vi "Caching_Expression_Evaluator_v4.vi"(0 "method":T1, 5 "variable":string, 7 "value in":dbl, 9 "expression/scriptlet":string, 11 "error in (no error)":errorcluster) -> (8 "value out":dbl, 15 "error out":errorcluster)   [LabVIEW 2013]
doc: "This \"object\" caches variables and parsed expressions for fast evaluation and assignment. It is possible to {set} or {get} a variable, {eval}uate an expression, or evaluate and {assign} an expression to a variable. The {isvalid} method tests whether a variable name is a valid identifier and does not collide with one of the predefined functions or numbers. To set initial values or define custom functions, {execute} a scriptlet.\n\nExpressions and scriptlets can make use Lua's arithmetic operators, the predefined numerical values \"pi\", \"_NaN\", and \"_Inf\", the functions in the math library (sin(), sqrt(), etc.) and the lv library functions for bitwise and other integer operations (andU32(), addI8(), etc.). To promote compact expressions, both sets of functions are available only without their library (\"math.\", \"lv.\") table prefix."
uses:
  t_Caching_Expression_Evaluator_Methods_v4.ctl
  LuaVIEW1.2.2_full_LV85/luaview/subvis/private/LuaVIEW Push (string).vi
  LuaVIEW1.2.2_full_LV85/luaview/subvis/private/LuaVIEW Push (number).vi
  LuaVIEW1.2.2_full_LV85/luaview/subvis/private/LuaVIEW Pull (number).vi
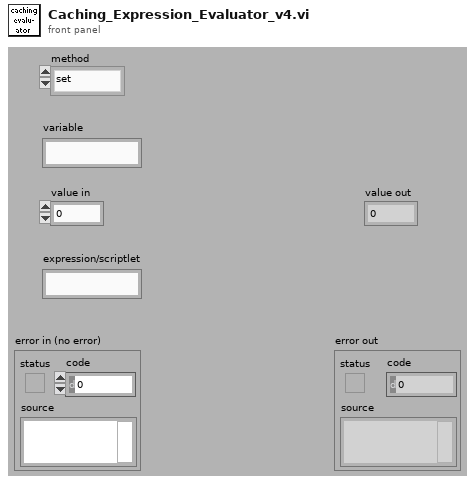
[diagram p1: front panel]
types:
  T1 = typedef "t_Caching_Expression_Evaluator_Methods_v4.ctl" = enum16{"set", "get", "eval", "eval2", "assign", "execute", "isvalid"}
  T2 = typedef "t_LuaVIEW Reference.ctl" = refnum<k1>
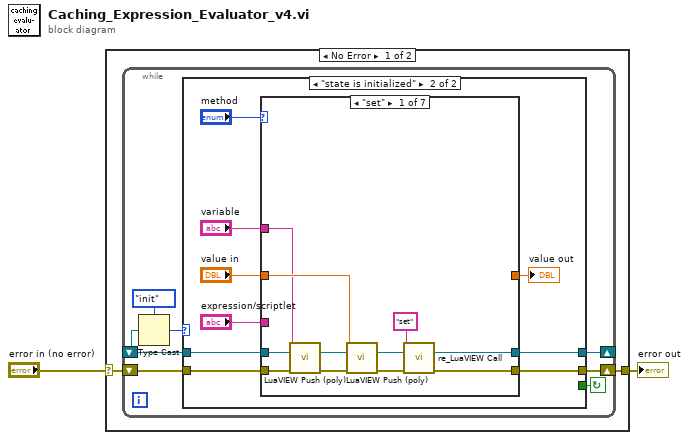
[diagram p0: block diagram]
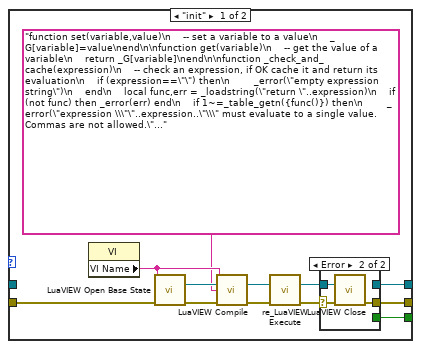
[diagram p2: hidden frame]
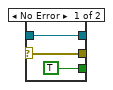
[diagram p3: hidden frame]
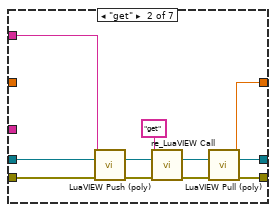
[diagram p4: hidden frame]
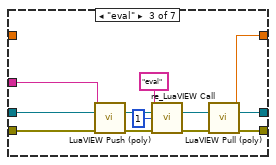
[diagram p5: hidden frame]
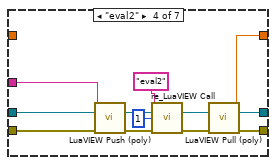
[diagram p6: hidden frame]
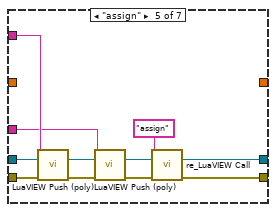
[diagram p7: hidden frame]
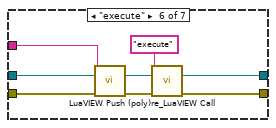
[diagram p8: hidden frame]
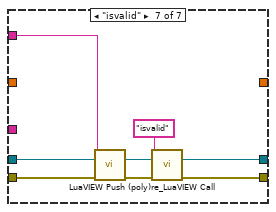
[diagram p9: hidden frame]
diagram:
  n1 = case shown="No Error" "error in (no error)" {
    selector: "error in (no error)" -> [w3 w112]
    tunnel: [w4 w112] -> w1
    frame No Error {
      n2 = while {
        shift-right: [w10] -> _
        shift-left: _ -> [w8]
        shift-right: [w9] -> w4
        shift-left: w3 -> [w11]
        stop <- w5 continue-if-true
        n3 = Type Cast(type=enum32{"init", "state is initialized"}."init", x=w8) -> (*(type *) &x=w6:enum32{"init", "state is initialized"})
        n4 = case shown="\"state is initialized\"" w6 {
          tunnel: w11 -> [w23 w38]
          tunnel: [w13 w35] -> w10
          tunnel: [w14 w36] -> w9
          tunnel: w8 -> [_ w37]
          tunnel: [w12 _] -> w5
          frame "init" {
            n5 = property class="VI"() -> ("VI Name"=w19:string)  [unwired: 2 in, 2 out]
            n6 = call "LuaVIEW Open Base State.vi"("close identifier (none)"=w19, "error in (no error)"=w23) -> ("LuaVIEW reference"=w21:T2, "error out"=w17:errorcluster)  [unwired: 12 out]
            n7 = call "LuaVIEW Compile.vi"("script name"=w19, "LuaVIEW reference in"=w21, "script"="function set(variable,value)\n    -- set a variable to a value\n    _G[variable]=value\nend\n\nfunction get(variable)\n    -- get the value of a variable\n    return _G[variable]\nend\n\nfunction _check_and_cache(expression)\n    -- check an expression, if OK cache it and return its evaluation\n    if (expression==\"\") then\n        _error(\"empty expression string\")\n    end\n    local func,err = _loadstring(\"return \"..expression)\n    if (not func) then _error(err) end\n    if 1~=_table_getn({func()}) then\n        _error(\"expression \\\"\"..expression..\"\\\" must evaluate to a single value. Commas are not allowed.\")\n    end\n    local result=func()\n    if _type(result)~=\"number\" then\n        _error(\"expression \\\"\"..expression..\"\\\" does not evaluate to a number\")\n    end\n    _expression_cache[expression]=func\n    return result\nend\n\nfunction eval(expression)\n    -- evaluate an expression and return its value\n    local func=_expression_cache[expression]\n    if (func) then\n        -- expression already parsed and cached\n        return func()\n    end\n    return _check_and_cache(expression)\nend\n\n-- New code from IBS\n-- Eval didn't work with my custom functions\nfunction eval2(expression)\n    -- evaluate an expression and return its value\n    local func=_expression_cache[expression]\n    if (not func) then\n        -- expression not parsed and cached\n        _check_and_cache(expression)\n        func=_expression_cache[expression]\n    end\n    -- expression is now parsed and cached\n    -- now make the desired tabular evaluation\n    \n    local answer;\n\n    dt = 0.1;\n    tMax = 1;\n    t = 0;\n    f = 0.1;\n    answer = func()\n    \n    return answer\nend\n\n\nfunction assign(variable,expression)\n    -- evaluate an expression and assign it to a variable\n    local func=_expression_cache[expression]\n    if (func) then\n        -- expression already parsed and cached\n        _G[variable]=func()\n        return\n    end\n    _G[variable]=_check_and_cache(expression)\nend\n\nfunction execute(statements)\n    -- execute statements, e.g. setting initial variable values\n    -- or defining custom functions\n    local func,err=_loadstring(statements)\n    if (not func) then\n        _error(err)\n    end\n    func()\nend\n\nfunction isvalid(variable)\n    -- check if a variable name is valid for assignment\n    if _name_reserved[variable] then\n        _error(\"\\\"\"..variable..\"\\\" is not a valid variable name: it is reserved for a predefined \".._type(_G[variable]))\n    end\n    if _string_find(variable,\"[^_%w]\") then\n        _error(\"\\\"\"..variable..\"\\\" is not a valid variable name: only underscores and alphanumerical characters are allowed.\")\n    end\n    if (not _loadstring(\"return {\"..variable..\"=42}\")) then\n        _error(\"\\\"\"..variable..\"\\\" is not a valid variable name: leading digits and Lua reserved names are prohibited.\")\n    end    \nend\n\n--start with an empty expression cache\n_expression_cache={}\n\n-- hide functions and tables that do not belong in expressions\n_error=error\n_type=type\n_table_getn=table.getn\n_string_find=string.find\n_loadstring=loadstring\nretain={\nretain=true,\nset=true,\nget=true,\neval=true,\nassign=true,\nexecute=true,\nisvalid=true,\nstring=true,\nmath=true,\n}\nfor k,v in pairs(lv) do\n    if (string.find(k,\"I8\") or string.find(k,\"U8\") or string.find(k,\"I16\") or string.find(k,\"U16\") or string.find(k,\"I32\") or string.find(k,\"U32\")) then\n        _G[k]=v\n        retain[k]=true\n    end\nend\n_name_reserved={}\nfor k,v in pairs(_G) do\n    if _type(k)==\"string\" and not (retain[k] or math[k] or string.sub(k,1,1)==\"_\") then\n        _G[k]=nil\n    else\n        _name_reserved[k]=true\n    end\nend\nmath=nil\n_name_reserved.math=nil\nretain=nil\n_name_reserved.retain=nil\nstring=nil\n_name_reserved.string=nil\n\nf=0\nt=0\ntMax = 0\ndt = 0", "error in (no error)"=w17) -> ("LuaVIEW reference out"=w20:T2, "error out"=w22:errorcluster)  [unwired: 10 out]
            n8 = call "re_LuaVIEW Execute.vi"("LuaVIEW reference in"=w20, "error in (no error)"=w22) -> ("LuaVIEW reference out"=w15:T2, "error out"=w16:errorcluster)  [unwired: 12 out]
            n9 = case shown="Error" w16 {
              selector: w16 -> [w25 w29]
              tunnel: w15 -> [w26 w28]
              tunnel: [w25 w27] -> w14
              tunnel: [w26 _] -> w13
              tunnel: [TRUE _] -> w12
              frame No Error {
              }
              frame Error {
                n10 = call "LuaVIEW Close.vi"("LuaVIEW reference"=w28, "error in (no error)"=w29) -> ("dup error"=w27:errorcluster)  [unwired: 13 out]
              }
            }
          }
          frame "state is initialized" {
            n11 = case shown="\"set\"" "method" {
              tunnel: w38 -> [w46 w50 w62 w74 w92 w99 w106]
              tunnel: w37 -> [w47 w51 w63 w75 w93 w100 w107]
              tunnel: [w39 w60 w72 w84 w85 w97 w104] -> w36
              tunnel: [w40 w55 w67 w79 w86 w98 w105] -> w35
              tunnel: "expression/scriptlet" -> [_ _ w64 w76 w87 w96 _]
              tunnel: "value in" -> [w42 _ _ _ _ _ _]
              tunnel: "variable" -> [w41 w52 _ _ w88 _ w108]
              tunnel: [_ w54 w66 w78 _ _ _] -> w30
              frame "set" {
                n12 = call-poly "LuaVIEW Push (poly).vi"("string"=w41, "LuaVIEW reference in"=w47, "error in (no error)"=w46) -> ("LuaVIEW reference out"=w44:T2, "error out"=w45:errorcluster)  [unwired: 11 out]
                n13 = call-poly "LuaVIEW Push (poly).vi"("number"=w42, "LuaVIEW reference in"=w44, "error in (no error)"=w45) -> ("LuaVIEW reference out"=w48:T2, "error out"=w49:errorcluster)  [unwired: 11 out]
                n14 = call "re_LuaVIEW Call.vi"("function name"="set", "LuaVIEW reference in"=w48, "error in (no error)"=w49) -> ("LuaVIEW reference out"=w40:T2, "error out"=w39:errorcluster)  [unwired: 11 out]
              }
              frame "get" {
                n15 = call-poly "LuaVIEW Push (poly).vi"("string"=w52, "LuaVIEW reference in"=w51, "error in (no error)"=w50) -> ("LuaVIEW reference out"=w58:T2, "error out"=w59:errorcluster)  [unwired: 11 out]
                n16 = call "re_LuaVIEW Call.vi"("function name"="get", "LuaVIEW reference in"=w58, "error in (no error)"=w59) -> ("LuaVIEW reference out"=w56:T2, "error out"=w57:errorcluster)  [unwired: 11 out]
                n17 = call-poly "LuaVIEW Pull (poly).vi"("LuaVIEW reference in"=w56, "error in (no error)"=w57) -> ("number"=w54:dbl, "LuaVIEW reference out"=w55:T2, "error out"=w60:errorcluster)  [unwired: 11 out]
              }
              frame "eval" {
                n18 = call-poly "LuaVIEW Push (poly).vi"("string"=w64, "LuaVIEW reference in"=w63, "error in (no error)"=w62) -> ("LuaVIEW reference out"=w70:T2, "error out"=w71:errorcluster)  [unwired: 11 out]
                n19 = call "re_LuaVIEW Call.vi"("function name"="eval", "LuaVIEW reference in"=w70, "required results (no checking needed)"=1, "error in (no error)"=w71) -> ("LuaVIEW reference out"=w68:T2, "error out"=w69:errorcluster)  [unwired: 10 out]
                n20 = call-poly "LuaVIEW Pull (poly).vi"("LuaVIEW reference in"=w68, "error in (no error)"=w69) -> ("number"=w66:dbl, "LuaVIEW reference out"=w67:T2, "error out"=w72:errorcluster)  [unwired: 11 out]
              }
              frame "eval2" {
                n21 = call-poly "LuaVIEW Push (poly).vi"("string"=w76, "LuaVIEW reference in"=w75, "error in (no error)"=w74) -> ("LuaVIEW reference out"=w82:T2, "error out"=w83:errorcluster)  [unwired: 11 out]
                n22 = call "re_LuaVIEW Call.vi"("function name"="eval2", "LuaVIEW reference in"=w82, "required results (no checking needed)"=1, "error in (no error)"=w83) -> ("LuaVIEW reference out"=w80:T2, "error out"=w81:errorcluster)  [unwired: 10 out]
                n23 = call-poly "LuaVIEW Pull (poly).vi"("LuaVIEW reference in"=w80, "error in (no error)"=w81) -> ("number"=w78:dbl, "LuaVIEW reference out"=w79:T2, "error out"=w84:errorcluster)  [unwired: 11 out]
              }
              frame "assign" {
                n24 = call-poly "LuaVIEW Push (poly).vi"("string"=w88, "LuaVIEW reference in"=w93, "error in (no error)"=w92) -> ("LuaVIEW reference out"=w90:T2, "error out"=w91:errorcluster)  [unwired: 11 out]
                n25 = call-poly "LuaVIEW Push (poly).vi"("string"=w87, "LuaVIEW reference in"=w90, "error in (no error)"=w91) -> ("LuaVIEW reference out"=w94:T2, "error out"=w95:errorcluster)  [unwired: 11 out]
                n26 = call "re_LuaVIEW Call.vi"("function name"="assign", "LuaVIEW reference in"=w94, "error in (no error)"=w95) -> ("LuaVIEW reference out"=w86:T2, "error out"=w85:errorcluster)  [unwired: 11 out]
              }
              frame "execute" {
                n27 = call-poly "LuaVIEW Push (poly).vi"("string"=w96, "LuaVIEW reference in"=w100, "error in (no error)"=w99) -> ("LuaVIEW reference out"=w102:T2, "error out"=w103:errorcluster)  [unwired: 11 out]
                n28 = call "re_LuaVIEW Call.vi"("function name"="execute", "LuaVIEW reference in"=w102, "error in (no error)"=w103) -> ("LuaVIEW reference out"=w98:T2, "error out"=w97:errorcluster)  [unwired: 11 out]
              }
              frame "isvalid" {
                n29 = call-poly "LuaVIEW Push (poly).vi"("string"=w108, "LuaVIEW reference in"=w107, "error in (no error)"=w106) -> ("LuaVIEW reference out"=w110:T2, "error out"=w111:errorcluster)  [unwired: 11 out]
                n30 = call "re_LuaVIEW Call.vi"("function name"="isvalid", "LuaVIEW reference in"=w110, "error in (no error)"=w111) -> ("LuaVIEW reference out"=w105:T2, "error out"=w104:errorcluster)  [unwired: 11 out]
              }
            }
            "value out" <- w30
          }
        }
      }
    }
    frame Error {
    }
  }
  "error out" <- w1
